vi "Find Specification Match.vi"(7 "error in (no error)":errorcluster, 8 "Channel List":string[](array[string]), 10 "file path (dialog if empty)":path) -> (0 "error out":errorcluster, 1 "IVI Specifications":string[][](array[string]), 3 "Channel Specs":string[][](array[string]))   [LabVIEW 2019]
uses:
  <vilib>/Utility/file.llb/Read Delimited Spreadsheet (string).vi
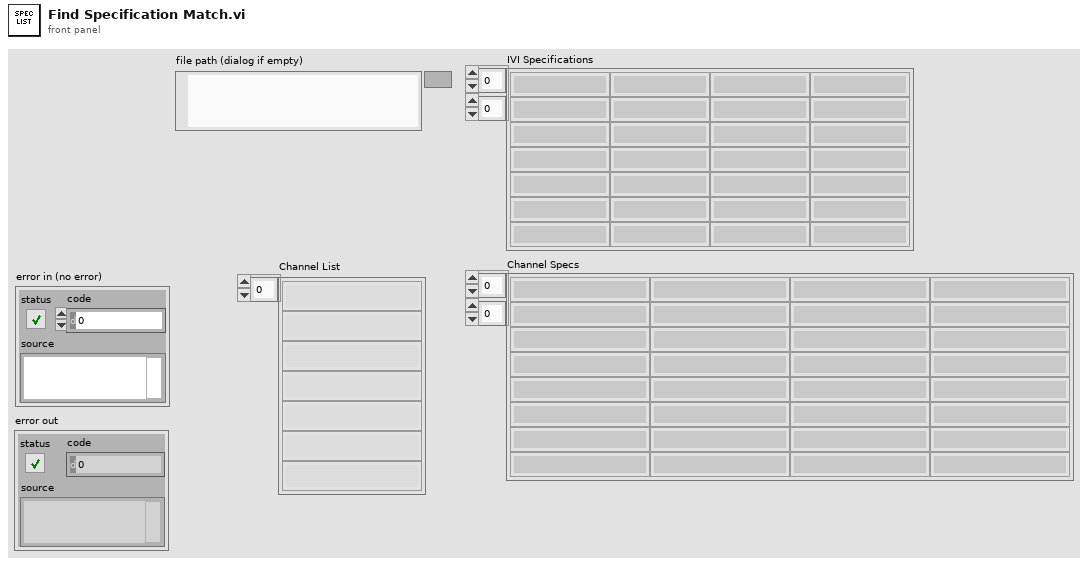
[diagram p1: front panel]
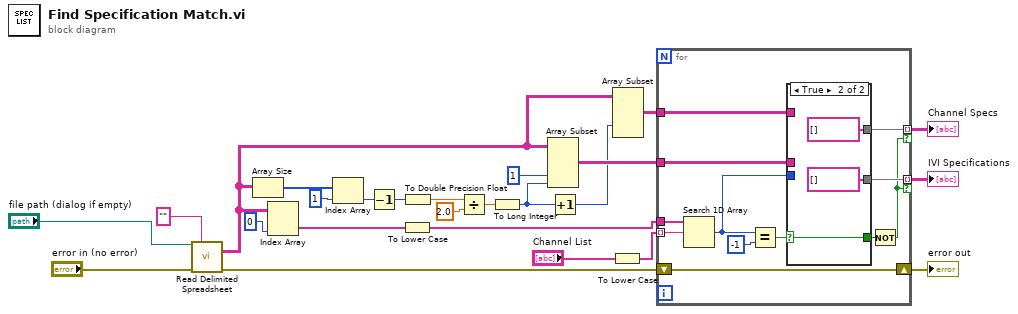
[diagram p0: block diagram]
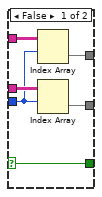
[diagram p2: hidden frame]
diagram:
  n1 = call-poly <vilib>:"Read Delimited Spreadsheet.vi"("file path (dialog if empty)"="file path (dialog if empty)", "format (%s)"="" ("format (%.3f)"), "error in (no error)"="error in (no error)") -> ("all rows"=w3:string[][], "error out"=w15:errorcluster)  [unwired: 7 in, 4 out]
  n2 = Array Size(array=w3) -> (size(s)=w14:i32[])
  n3 = Index Array(array=w3, index (col)=0 ("disabled index (col)")) -> (element=w1:string[])  [unwired: 1 in]
  n4 = Index Array(array=w14, index=1) -> (element=w12:i32)
  n5 = Decrement(x=w12) -> (x-1=w11:i32)
  n6 = To Lower Case(string=w1) -> (all lower case string=w4:string[])
  n7 = To Double Precision Float(number=w11) -> (double precision float=w7:dbl)
  n8 = Divide(x=w7, y=2.0) -> (x/y=w10:dbl)
  n9 = To Long Integer(number=w10) -> (32bit integer=w9:i32)
  n10 = Array Subset(array=w3, index (col)=1 ("index"), length (col)=w9) -> (w19:string[][])  [unwired: 2 in]
  n11 = Increment(x=w9) -> (x+1=w8:i32)
  n12 = To Lower Case(string="Channel List") -> (all lower case string=w5:string[])
  n13 = Array Subset(array=w3, index (col)=w8) -> (w20:string[][])  [unwired: 3 in]
  n14 = for {
    tunnel: w5 -> [w37] mode=indexing
    tunnel: w20 -> [w36]
    tunnel: [w35] -> w18 mode=indexing if=w26
    tunnel: w19 -> [w34]
    tunnel: [w29] -> w17 mode=indexing if=w26
    tunnel: w4 -> [w27]
    shift-right: [w33] -> w16
    shift-left: w15 -> [w33]
    n15 = Search 1D Array(1D array=w27, element=w37) -> (index of element=w32:i32)  [unwired: 1 in]
    n16 = Equal?(x=w32, y=-1) -> (x = y?=w30:bool)
    n17 = case shown="True" w30 {
      selector: w30 -> [w38 w44]
      tunnel: w36 -> [w43 _]
      tunnel: [w42 string[] []] -> w35
      tunnel: w34 -> [w41 _]
      tunnel: [w40 string[] []] -> w29
      tunnel: w32 -> [w39 _]
      tunnel: [w38 w44] -> w28
      frame False {
        n18 = Index Array(array=w43, index (row)=w39) -> (element=w42:string[])  [unwired: 1 in]
        n19 = Index Array(array=w41, index (row)=w39) -> (element=w40:string[])  [unwired: 1 in]
      }
      frame True {
      }
    }
    n20 = Not(x=w28) -> (.not. x?=w26:bool)
  }
  "Channel Specs" <- w18
  "IVI Specifications" <- w17
  "error out" <- w16
